vi "Init.vi"(8 "error in (no error)":errorcluster, 11 "Token":string) -> (0 "error out":errorcluster, 3 "NCDC Weather out":refnum<class "NCDC Weather.lvclass">)   [LabVIEW 2020, in "NCDC Weather.lvclass"]
uses:
  NCDC Weather.lvclass
  NCDC Weather.lvclass/NCDC Weather.ctl
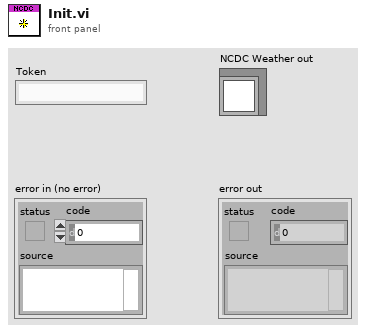
[diagram p1: front panel]
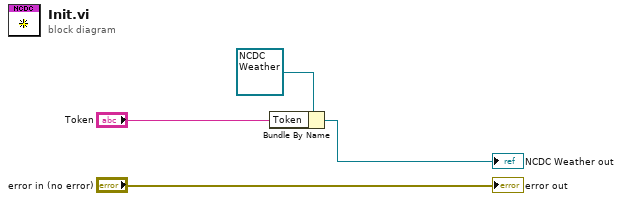
[diagram p0: block diagram]
diagram:
  n1 = Bundle By Name(cluster=refnum<class "NCDC Weather.lvclass"> refnum ("NCDC Weather in"), "Token"="Token") -> (→"NCDC Weather out":refnum<class "NCDC Weather.lvclass">)
  "error out" <- "error in (no error)"
